vi "HT_add.vi"(8 "input valid":bool=TRUE, 10 "y":fxp<+/-,16,14>, 11 "x":fxp<+/-,16,14>) -> (0 "output valid":bool, 3 "x+y":fxp<+/-,16,14>)   [LabVIEW 2013]
uses:
  <vilib>/rvi/FXPMathLib/FxpConvert/subVIs/nifxpmath_Convert_SimConfig.ctl
  <vilib>/fxp/LVFixedPointQuantizationPolicyTypeDef.ctl
  <vilib>/fxp/LVFixedPointOverflowPolicyTypeDef.ctl
  <vilib>/rvi/FXPMathLib/FxpConvert/simVIs/DllFxpConvertTemp_sub.vi
  <vilib>/rvi/FXPMathLib/FxpConvert/XNode/nifxpmath_Convert.xnode
  <vilib>/rvi/FXPMathLib/FxpAdd/XNode/nifxpmath_Add.xnode
  <vilib>/rvi/FXPMathLib/sim/FxpSim.dll
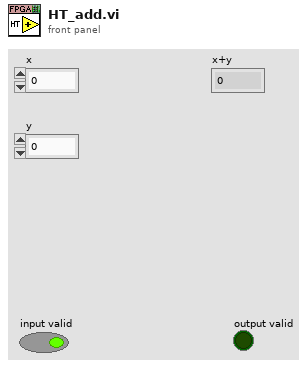
[diagram p1: front panel]
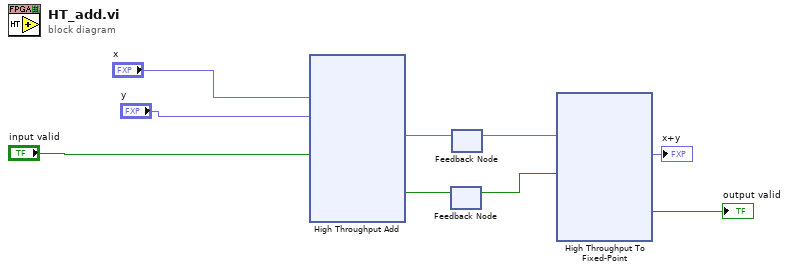
[diagram p0: block diagram]
diagram:
  n1 = xnode "High Throughput Add"("x"="x", "y"="y", "input valid"="input valid") -> ("x+y"=w9:fxp<+/-,17,15>, "output valid"=w4:bool)  [unwired: 1 in, 1 out]
  n2 = feedback #1() -> (w7:bool)  [unwired: 1 in]
  n3 = feedback-in #1(w4) -> ()
  n4 = feedback #2() -> (w8:fxp<+/-,17,15>)  [unwired: 1 in]
  n5 = feedback-in #2(w9) -> ()
  n6 = xnode "High Throughput To Fixed-Point"("x"=w8, "input valid"=w7) -> ("y"=→"x+y":fxp<+/-,16,14>, "output valid"=→"output valid":bool)  [unwired: 1 in, 1 out]
